vi "Kill Job.vi"(8 "error in (no error)":errorcluster, 11 "Job in":refnum<class "Job.lvclass">) -> (0 "error out":errorcluster, 3 "Job out":refnum<class "Job.lvclass">)   [LabVIEW 2013, in "openCronJob.lvlib" / "Job.lvclass"]
uses:
  Job.lvclass
  Job.lvclass/Job.ctl
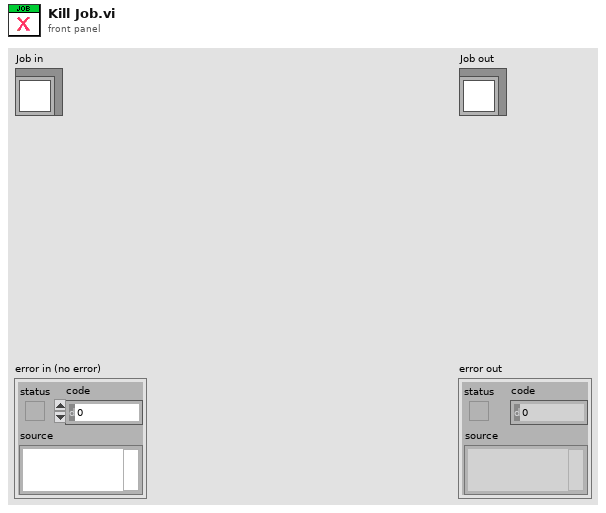
[diagram p1: front panel]
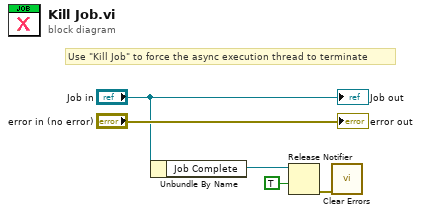
[diagram p0: block diagram]
diagram:
  # "Use \"Kill Job\" to force the async execution thread to terminate"
  n1 = Unbundle By Name("Job in") -> ("Job Complete"=w3:refnum<notifier>)
  n2 = Release Notifier(notifier=w3, force destroy? (F)=TRUE) -> (error out=w2:errorcluster)  [unwired: 1 in, 2 out]
  n3 = call <vilib>:"Clear Errors.vi"("error in (no error)"=w2) -> ()  [unwired: 6 in, 1 out]
  "error out" <- "error in (no error)"
  "Job out" <- "Job in"
